vi "Generate Report.vi"(8 "error in (no error)":errorcluster, 10 "Resource In":variant, 11 "HIJ IMAQdx Display in":refnum<class "HIJ IMAQdx Display.lvclass">) -> (0 "error out":errorcluster, 2 "Resource Out":variant, 3 "HIJ IMAQdx Display out":refnum<class "HIJ IMAQdx Display.lvclass">)   [LabVIEW 2020, in "HIJ IMAQdx Display.lvlib" / "HIJ IMAQdx Display.lvclass"]
uses:
  HIJ IMAQdx Display.lvclass
  HIJ IMAQdx Display.lvclass/HIJ IMAQdx Display.ctl
  <vilib>/Utility/config.llb/NI_LVConfig.lvlib
  <vilib>/Utility/config.llb/Write Key (Boolean).vi
  <vilib>/Utility/config.llb/Config Data RefNum.ctl
  HIJ Vision Display/HIJ Vision Display/HIJ Vision Display.lvclass
  Camera Actors/IMAQdx Actor/IMAQdx Actor/IMAQdx Actor.lvclass
  <vilib>/Utility/config.llb/Write Key (Double).vi
  <vilib>/Utility/config.llb/Write Key (String).vi
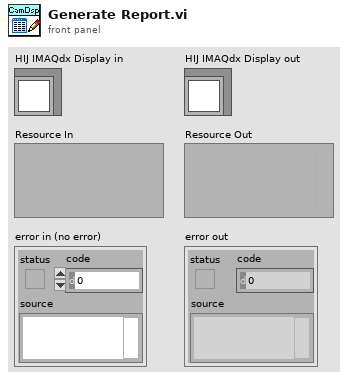
[diagram p1: front panel]
types:
  T1 = typedef "NI_LVConfig.lvlib/Config Data RefNum.ctl" = refnum<k1>
  T2 = typedef "IMAQ Image.ctl" = refnum<image>
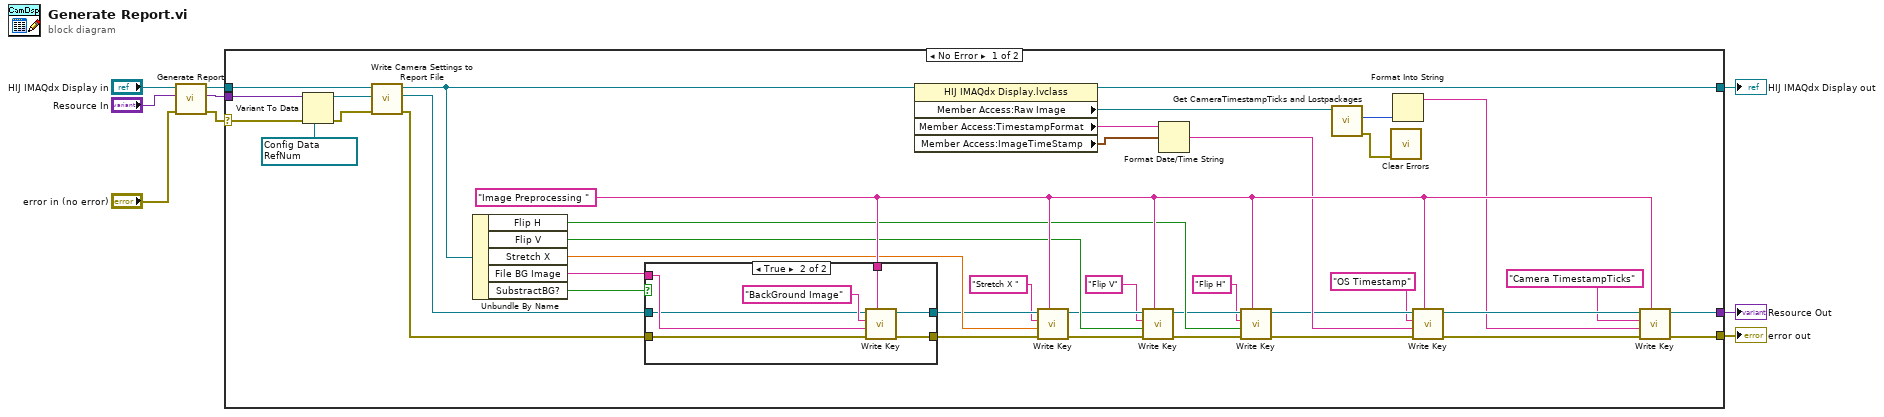
[diagram p0: block diagram]
diagram:
  n1 = call-parent "Generate Report.vi"("error in (no error)"="error in (no error)", "Resource In"="Resource In", "HIJ Vision Display in"="HIJ IMAQdx Display in") -> ("error out"=w9:errorcluster, "Resource Out"=w4:variant, "HIJ Vision Display out"=w8:refnum<class "HIJ IMAQdx Display.lvclass">)  [unwired: 6 in]
  n2 = case shown="No Error" w9 {
    selector: w9 -> [w46 w60]
    tunnel: w4 -> [w47 w61]
    tunnel: [w15 w60] -> w3
    tunnel: [w18 w61] -> w2
    tunnel: [w23 w59] -> w1
    tunnel: w8 -> [w45 w59]
    frame No Error {
      w29 = T1 refnum items=["config data"] ("refnum out")
      w49 = "Image Preprocessing " ("section")
      n3 = Variant To Data(error in=w46, type=w29, Variant=w47) -> (data=w27:T1, error out=w26:errorcluster)
      n4 = call-dynamic "Write Camera Settings to Report File.vi"("error in (no error)"=w26, "refnum in"=w27, "HIJ IMAQdx Display in"=w45) -> ("error out"=w25:errorcluster, "refnum out"=w24:T1, "HIJ IMAQdx Display out"=w28:refnum<class "HIJ IMAQdx Display.lvclass">)  [unwired: 6 in]
      n5 = Unbundle By Name(w28) -> ("Flip H"=w40:bool, "Flip V"=w41:bool, "Stretch X"=w42:dbl, "File BG Image"=w43:string, "SubstractBG?"=w30:bool)
      n6 = case shown="True" w30 {
        tunnel: w25 -> [w51 w58]
        tunnel: w43 -> [_ w57]
        tunnel: [w50 w56] -> w39
        tunnel: [w51 w55] -> w38
        tunnel: w49 -> [_ w53]
        tunnel: w24 -> [w50 w52]
        frame False {
        }
        frame True {
          n7 = call-poly <vilib>:"Write Key.vi"("section"=w53, "error in (no error)"=w58, "value"=w57, "key"="BackGround Image" ("section"), "refnum"=w52) -> ("error out"=w55:errorcluster, "refnum out"=w56:T1)  [unwired: 4 in, 1 out]
        }
      }
      n8 = property class="HIJ IMAQdx Display.lvclass"(reference=w28) -> (reference out=w23:refnum<class "HIJ IMAQdx Display.lvclass">, "Member Access:Raw Image"=w22:T2, "Member Access:TimestampFormat"=w21:string, "Member Access:ImageTimeStamp"=w20:timestamp)  [unwired: 1 in, 1 out]
      n9 = call-poly <vilib>:"Write Key.vi"("section"=w49, "error in (no error)"=w38, "value"=w42, "key"="Stretch X " ("section"), "refnum"=w39) -> ("error out"=w36:errorcluster, "refnum out"=w37:T1)  [unwired: 4 in, 1 out]
      n10 = call-poly <vilib>:"Write Key.vi"("section"=w49, "error in (no error)"=w36, "value"=w41, "key"="Flip V" ("section"), "refnum"=w37) -> ("error out"=w34:errorcluster, "refnum out"=w35:T1)  [unwired: 4 in, 1 out]
      n11 = Format Date/Time String(time format string (%c)=w21, seconds (now)=w20) -> (date/time string=w48:string)  [unwired: 1 in]
      n12 = call-poly <vilib>:"Write Key.vi"("section"=w49, "error in (no error)"=w34, "value"=w40, "key"="Flip H" ("section"), "refnum"=w35) -> ("error out"=w14:errorcluster, "refnum out"=w44:T1)  [unwired: 4 in, 1 out]
      n13 = call "Get CameraTimestampTicks and Lostpackages.vi"("image in"=w22) -> ("error out"=w17:errorcluster, "CameraTimestampTicks"=w11:u64)  [unwired: 7 in, 2 out]
      n14 = call <vilib>:"Clear Errors.vi"("error in (no error)"=w17) -> ()  [unwired: 5 in, 2 out]
      n15 = Format Into String(w11) -> (resulting string=w10:string)  [unwired: 3 in, 1 out]
      n16 = call-poly <vilib>:"Write Key.vi"("section"=w49, "error in (no error)"=w14, "value"=w48, "key"="OS Timestamp" ("section"), "refnum"=w44) -> ("error out"=w13:errorcluster, "refnum out"=w19:T1)  [unwired: 4 in, 1 out]
      n17 = call-poly <vilib>:"Write Key.vi"("section"=w49, "error in (no error)"=w13, "value"=w10, "key"="Camera TimestampTicks" ("section"), "refnum"=w19) -> ("error out"=w15:errorcluster, "refnum out"=w18:T1)  [unwired: 4 in, 1 out]
    }
    frame Error {
    }
  }
  "error out" <- w3
  "HIJ IMAQdx Display out" <- w1
  "Resource Out" <- w2
